vi "mod_Narrow band low pass filter design (multistage).vi"(0 "Maximum Decimation Factor (512)":enum16{"512", "1024", "2048", "4096"}(ring), 5 "Stop Band Attenuation (120 dB)":T1(ring)=enum."120 dB", 12 "Alias Protect in Final Transition? (T)":bool=TRUE) -> (4 "Filter Info":cluster{"h":dbl[], "Decimation":dbl} {"h" format="%.2f"; "Decimation" format="%.2f"})   [LabVIEW 2020, in "niAMT.lvlib"]
uses:
  <vilib>/addons/Modulation/niAMT.lvlib
  <vilib>/Analysis/2dsp.llb/1D Convolution (DBL).vi
  <vilib>/Analysis/NI_AALPro.lvlib
  <vilib>/measure/NI_MAPro.lvlib
panel:
  in  "debug?":bool
  out "frequency response":cluster{"Mag H(w)":dbl[]}[](graph)
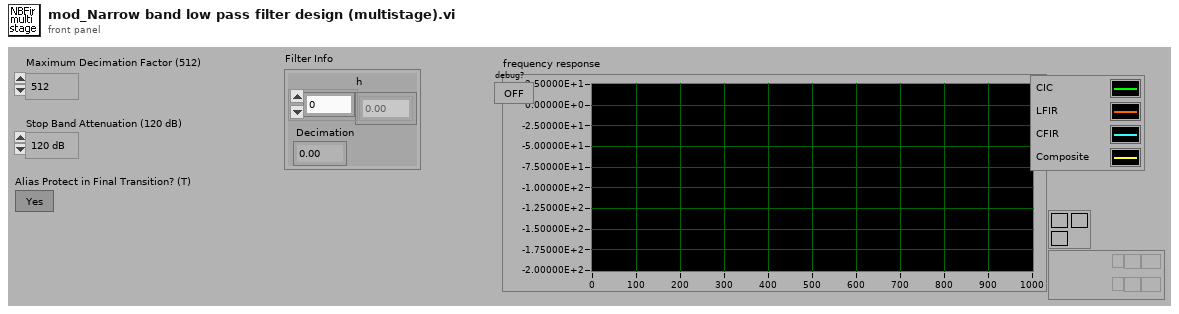
[diagram p1: front panel]
types:
  T1 = enum16{"48 dB", "60 dB", "72 dB", "84 dB", "96 dB", "120 dB"}
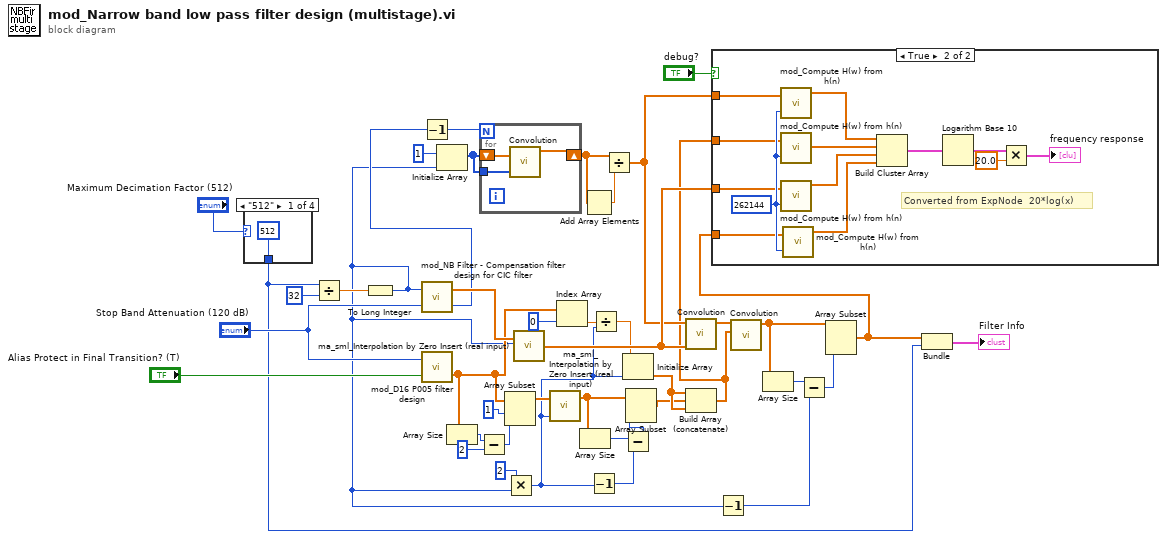
[diagram p0: block diagram]
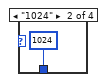
[diagram p3: hidden frame]
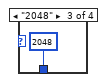
[diagram p4: hidden frame]
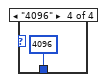
[diagram p5: hidden frame]
diagram:
  n1 = case shown="\"512\"" "Maximum Decimation Factor (512)" {
    tunnel: [512 1024 2048 4096] -> w2
    frame "512" {
    }
    frame "1024" {
    }
    frame "2048" {
    }
    frame "4096" {
    }
  }
  n2 = Divide(x=w2, y=32) -> (x/y=w40:dbl)
  n3 = To Long Integer(number=w40) -> (32bit integer=w7:i32)
  n4 = call <vilib>:"mod_NB Filter - Compensation filter design for CIC filter.vi"("stop band attenuation"="Stop Band Attenuation (120 dB)", "M"=w7) -> ("CIC stages"=w35:i32, "filter coefficients"=w38:dbl[])
  n5 = Decrement(x=w35) -> (x-1=w34:i32)
  n6 = call <vilib>:"mod_D16 P005 filter design.vi"("alias protect in final transition"="Alias Protect in Final Transition? (T)", "stop band attenuation"="Stop Band Attenuation (120 dB)") -> ("h"=w20:dbl[])
  n7 = Initialize Array(1, w7) -> (w33:i32[])
  n8 = Array Size(array=w20) -> (size(s)=w24:i32)
  n9 = Subtract(x=w24, y=2) -> (x-y=w25:i32)
  n10 = for {
    N: w34 -> [_]
    shift-right: [w47] -> w32
    shift-left: w33 -> [w49]
    tunnel: w33 -> [w48]
    n11 = call-poly <vilib>:"Convolution.vi"("Y"=w48, "X"=w49) -> ("X * Y"=w47:dbl[])  [unwired: 1 in, 8 out]
  }
  n12 = Array Subset(array=w20, index=1 ("Array Index"), length=w25) -> (w16:dbl[])
  n13 = Multiply(x=2, y=w7) -> (x*y=w5:i32)
  n14 = call <vilib>:"ma_sml_Interpolation by Zero Insert (real input).vi"("L"=w7, "x"=w38) -> ("y"=w29:dbl[])
  n15 = call <vilib>:"ma_sml_Interpolation by Zero Insert (real input).vi"("L"=w5, "x"=w16) -> ("y"=w11:dbl[])
  n16 = Index Array(array=w20, index=0 ("Index")) -> (element=w21:dbl)
  n17 = Array Size(array=w11) -> (size(s)=w10:i32)
  n18 = Add Array Elements(numeric array=w32) -> (sum=w31:dbl)
  n19 = Decrement(x=w5) -> (x-1=w8:i32)
  n20 = Divide(x=w21, y=w5) -> (x/y=w14:dbl)
  n21 = Divide(x=w32, y=w31) -> (x/y=w28:dbl[])
  n22 = Initialize Array(w14, w5) -> (w13:dbl[])
  n23 = Subtract(x=w10, y=w8) -> (x-y=w9:i32)
  n24 = Array Subset(array=w11, length=w9) -> (w12:dbl[])  [unwired: 1 in]
  n25 = call-poly <vilib>:"Convolution.vi"("Y"=w29, "X"=w28) -> ("X * Y"=w26:dbl[])  [unwired: 1 in, 8 out]
  n26 = Build Array (concatenate)(w13, w12, w13) -> (w15:dbl[])
  n27 = Decrement(x=w7) -> (x-1=w6:i32)
  n28 = call-poly <vilib>:"Convolution.vi"("Y"=w15, "X"=w26) -> ("X * Y"=w19:dbl[])  [unwired: 1 in, 8 out]
  n29 = Array Size(array=w19) -> (size(s)=w18:i32)
  n30 = Subtract(x=w18, y=w6) -> (x-y=w17:i32)
  n31 = Array Subset(array=w19, length=w17) -> (w3:dbl[])  [unwired: 1 in]
  n32 = case shown="True" "debug?" {
    tunnel: w29 -> [_ w57]
    tunnel: w28 -> [_ w56]
    tunnel: w15 -> [_ w55]
    tunnel: w3 -> [_ w54]
    frame False {
    }
    frame True {
      w59 = 262144 ("FFT size")
      # "Converted from ExpNode \t20*log(x)"
      n33 = call <vilib>:"mod_Compute H(w) from h(n).vi"("h"=w56, "FFT size"=w59) -> ("Mag H(w)"=w62:dbl[])  [unwired: 2 out]
      n34 = call <vilib>:"mod_Compute H(w) from h(n).vi"("h"=w55, "FFT size"=w59) -> ("Mag H(w)"=w61:dbl[])  [unwired: 2 out]
      n35 = call <vilib>:"mod_Compute H(w) from h(n).vi"("h"=w57, "FFT size"=w59) -> ("Mag H(w)"=w60:dbl[])  [unwired: 2 out]
      n36 = call <vilib>:"mod_Compute H(w) from h(n).vi"("h"=w54, "FFT size"=w59) -> ("Mag H(w)"=w58:dbl[])  [unwired: 2 out]
      n37 = Build Cluster Array(w62, w61, w60, w58) -> (w51:cluster{"Mag H(w)":dbl[]}[])
      n38 = Logarithm Base 10(1:w51) -> (0:w52:cluster{"Mag H(w)":dbl[]}[])
      n39 = Multiply(x=w52, y=20.0) -> (x*y=→"frequency response":cluster{"Mag H(w)":dbl[]}[])
    }
  }
  n40 = Bundle(w3, w2) -> (→"Filter Info":cluster{dbl[], i32})  [unwired: 1 out]
